vi "VI Tree.vi"   [LabVIEW 2017, in "RadWag balances and scales.lvlib"]
doc: "This is the instrument driver for the Balances manufactured by Radwag. The VI Tree displays all the user-callable VIs of the instrument driver in an organized table."
uses:
  <instrlib>/Radwag Balances and Scales/Public/RadWag balances and scales.lvlib
panel:
  # "(c) 2014 Przemysłowy Instytut Automatyki i Pomiarów PIAP.  ALL RIGHTS RESERVED."
  # "SEE DIAGRAM\nFOR VI TREE."
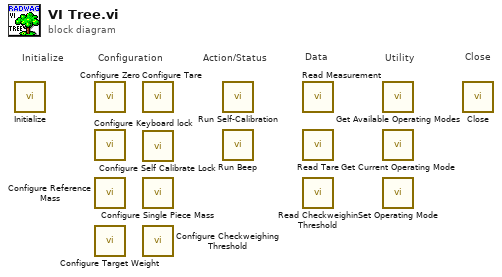
[diagram p0: block diagram]
diagram:
  # "Close"
  # "Configuration"
  # "Utility"
  # "Data"
  # "Action/Status"
  # "Initialize"
  n1 = call <instrlib>:"Initialize.vi"() -> ()  [unwired: 10 in, 2 out]
  n2 = call <instrlib>:"Configure Zero.vi"() -> ()  [unwired: 10 in, 2 out]
  n3 = call <instrlib>:"Configure Keyboard lock.vi"() -> ()  [unwired: 10 in, 2 out]
  n4 = call <instrlib>:"Configure Reference Mass.vi"() -> ()  [unwired: 10 in, 2 out]
  n5 = call <instrlib>:"Configure Target Weight.vi"() -> ()  [unwired: 10 in, 2 out]
  n6 = call <instrlib>:"Configure Tare.vi"() -> ()  [unwired: 10 in, 2 out]
  n7 = call <instrlib>:"Configure Self Calibrate Lock.vi"() -> ()  [unwired: 10 in, 2 out]
  n8 = call <instrlib>:"Configure Single Piece Mass.vi"() -> ()  [unwired: 10 in, 2 out]
  n9 = call <instrlib>:"Configure Checkweighing Threshold.vi"() -> ()  [unwired: 10 in, 2 out]
  n10 = call <instrlib>:"Run Self-Calibration.vi"() -> ()  [unwired: 9 in, 3 out]
  n11 = call <instrlib>:"Run Beep.vi"() -> ()  [unwired: 8 in, 4 out]
  n12 = call <instrlib>:"Read Measurement.vi"() -> ()  [unwired: 7 in, 5 out]
  n13 = call <instrlib>:"Read Tare.vi"() -> ()  [unwired: 8 in, 4 out]
  n14 = call <instrlib>:"Read Checkweighin Threshold.vi"() -> ()  [unwired: 8 in, 4 out]
  n15 = call <instrlib>:"Get Available Operating Modes.vi"() -> ()  [unwired: 9 in, 3 out]
  n16 = call <instrlib>:"Get Current Operating Mode.vi"() -> ()  [unwired: 9 in, 3 out]
  n17 = call <instrlib>:"Set Operating Mode.vi"() -> ()  [unwired: 10 in, 2 out]
  n18 = call <instrlib>:"Close.vi"() -> ()  [unwired: 11 in, 1 out]
